vi "Autosize Listbox Columns (Uniform Text) Table UT.vi"(4 "error in (no error)":errorcluster, 5 "extra padding (0)":i16, 6 "max width (px)":i16, 7 "Table ref":refnum<vi>) -> (0 "error out":errorcluster, 3 "Table ref":refnum<vi>)   [LabVIEW 2019, in "Sports Unit Tests.lvclass"]
doc: "This VI resizes each column of the table specified by Table Ref based on the widest entry of the column. Additionally, if Resize Table? is TRUE, the VI will set the table width based on the number of populated columns."
uses:
  Sports Unit Tests.lvclass
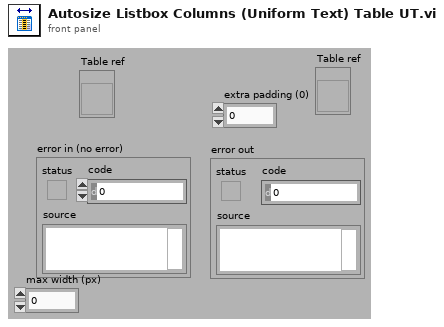
[diagram p1: front panel]
types:
  T1 = enum16{"User-specified Font", "Application Font", "System Font", "Dialog Font"}
  T2 = cluster{"Font Name:":string, "Size":i16, "Strikeout?":bool, "Italic?":bool, "Underline?":bool, "Outline?":bool, "Shadow?":bool, "Bold?":bool}
  T3 = cluster{"left":i16, "top":i16, "right":i16, "bottom":i16}
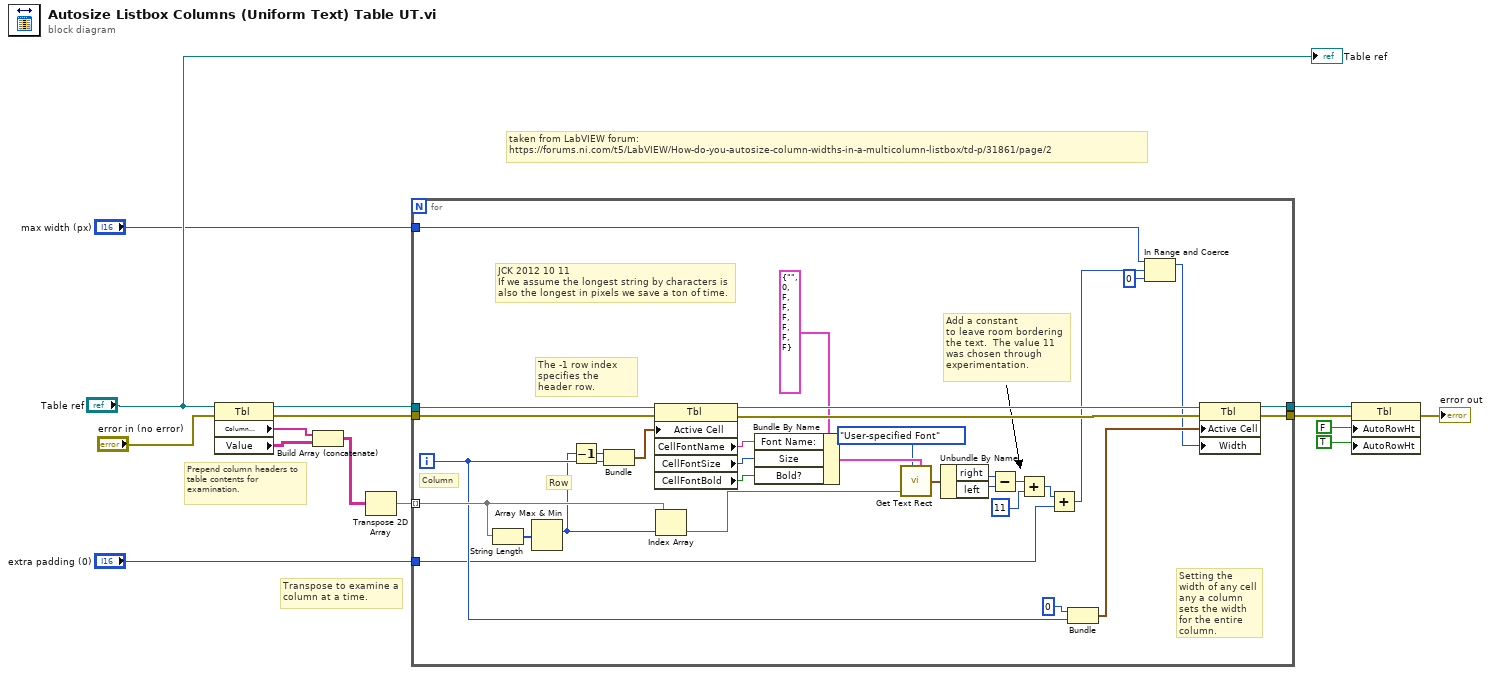
[diagram p0: block diagram]
diagram:
  # "taken from LabVIEW forum:\nhttps://forums.ni.com/t5/LabVIEW/How-do-you-autosize-column-widths-in-a-multicolumn-listbox/td-p/31861/page/2"
  # "Transpose to examine a column at a time."
  # "Prepend column headers to table contents for examination."
  n1 = property class="Tbl"(reference="Table ref", error in="error in (no error)") -> (reference out=w15:refnum<vi>, error out=w11:errorcluster, "Column Headers[]"=w14:string[], "Value"=w10:string[][])
  n2 = Build Array (concatenate)(w14, w10) -> (w13:string[][])
  n3 = Transpose 2D Array(2D array=w13) -> (transposed array=w12:string[][])
  n4 = for {
    tunnel: w12 -> [w47] mode=indexing
    tunnel: w15 -> [w46]
    tunnel: w11 -> [w45]
    tunnel: [w40] -> w3
    tunnel: [w39] -> w4
    tunnel: "extra padding (0)" -> [w37]
    tunnel: "max width (px)" -> [w18]
    i -> [w38]
    # "JCK 2012 10 11\nIf we assume the longest string by characters is also the longest in pixels we save a ton of time."
    # "The -1 row index specifies the header row."
    # "Add a constant\nto leave room bordering the text.  The value 11 was chosen through experimentation."
    # "Row"
    # "Setting the width of any cell any a column sets the width for the entire column."
    # "Column"
    n5 = String Length(string=w47) -> (length=w36:i32[])
    n6 = Array Max & Min(array=w36) -> (max index (indices)=w22:i32)  [unwired: 3 out]
    n7 = Decrement(x=w22) -> (x-1=w32:i32)
    n8 = Bundle(w32, w38) -> (w23:cluster{i32, i32})  [unwired: 1 in]
    n9 = property class="Tbl"(reference=w46, error in=w45, "Active Cell"=w23) -> (reference out=w44:refnum<vi>, error out=w43:errorcluster, "CellFontName"=w25:string, "CellFontSize"=w34:u32, "CellFontBold"=w26:bool)
    n10 = Index Array(array=w47, index=w22) -> (element=w21:string)
    n11 = Bundle By Name(cluster=T2 {"Font Name:"="", "Size"=0, "Strikeout?"=FALSE, "Italic?"=FALSE, "Underline?"=FALSE, "Outline?"=FALSE, "Shadow?"=FALSE, "Bold?"=FALSE} ("[user-specified font]"), "Font Name:"=w25, "Size"=w34, "Bold?"=w26) -> (w28:T2)
    n12 = call <vilib>:"Get Text Rect.vi"("desired font(Application)"=T1."User-specified Font", "text"=w21, "[user-specified font]"=w28) -> ("rect"=w29:T3)  [unwired: 6 in]
    n13 = Unbundle By Name(w29) -> ("right"=w30:i16, "left"=w31:i16)
    n14 = Subtract(x=w30, y=w31) -> (x-y=w33:i16)
    n15 = Add(x=w33, y=i16 11) -> (x+y=w20:i16)
    n16 = Add(x=w20, y=w37) -> (x+y=w19:i16)
    n17 = Bundle(0, w38) -> (w41:cluster{i32, i32})  [unwired: 1 in]
    n18 = In Range and Coerce(upper limit=w18, x=w19, lower limit=i16 0) -> (coerced(x)=w16:i16)  [unwired: 1 out]
    n19 = property class="Tbl"(reference=w44, error in=w43, "Active Cell"=w41, "Width"=w16) -> (reference out=w39:refnum<vi>, error out=w40:errorcluster)
  }
  n20 = property class="Tbl"(reference=w4, error in=w3, "AutoRowHt"=FALSE ("Autosizing Row Height"), "AutoRowHt"=TRUE ("Autosizing Row Height")) -> (error out=→"error out":errorcluster)  [unwired: 1 out]
  "Table ref" <- "Table ref"
